vi "Trav_pos_global.vi"() -> ()   [LabVIEW 2010]
uses:
  Gen Trav/Traverse_cluster.ctl
  Gen Trav/Spacing.ctl
  Controls/Multi_run_mode.ctl
  Controls/Tunnel_Coordinates.ctl
panel:
  in  "Repeat Rows?":bool
  in  "Pause Until Seconds 1904":dbl
  in  "FFID Background":T1 {"Row Duration (mins)" format="%#.1f"; "Row No" min=0; "Trace Gas Concentration (%)" min=0.0 format="%#.2f"; "Emission Rate (l/min)" format="%#.2f"; "Tunnel Speed" format="%#.2f"; "Start X" format="%#.2f"; "Start Y" format="%#.2f"; "Start Z" format="%#.2f"; "End X" format="%#.2f"; "End Y" format="%#.2f"; "End Z" format="%#.2f"; "Averaging time (min)" min=0.0 format="%#.1f"}
  in  "Meas Setup Number":i32
  in  "Current Meas Setup File":string
  in  "Default Traverse Setup":string
  out "Simulation Time":timestamp
  out "Row completion times":timestamp[](array[timestamp])
  in  "Dummy Measurement?":bool
  in  "Jumped Positions":dbl[][](array[numeric])
  in  "Jump Bad Positions?":bool
  in  "Model Rotation (deg)":dbl format="%.2f"
  in  "Work in Tunnel Coordinates?":T4
  in  "Show User Metadata on Launch?":bool=TRUE
  in  "Measurement setup files":string[](array[string])
  out "Live Traverse Preview?":bool
  in  "Paused During Row?":bool
  in  "Speed Factor":dbl=1.0 min=0.1 max=5.0 format="%.2f"
  in  "Estimated Completion time":string
  in  "Start of Row time (Sec)":dbl
  out "Currently on point":i32=9
  in  "Current Row":T1 {"Row Duration (mins)" format="%#.1f"; "Row No" min=0; "Trace Gas Concentration (%)" min=0.0 format="%#.2f"; "Emission Rate (l/min)" format="%#.2f"; "Tunnel Speed" format="%#.2f"; "Start X" format="%#.2f"; "Start Y" format="%#.2f"; "Start Z" format="%#.2f"; "End X" format="%#.2f"; "End Y" format="%#.2f"; "End Z" format="%#.2f"; "Averaging time (min)" min=0.0 format="%#.1f"}
  in  "Source Control?":bool
  in  "Top level setup filename":path
  in  "Pause Acquisition":bool
  out "Axis Traversed":enum16{"X traverse", "Y traverse", "Z traverse"}(ring)
  in  "Traverse position":dbl[](array[numeric])=[0.0, 0.0, 0.0] format="%.2f"
  in  "Present Probe Positions":T5(array[cluster]) {"Z" format="%.1f"; "Y" format="%.1f"; "X" format="%.1f"}
  # "X                Y                   Z"
  # "X           Y            Z"
  # "Start"
  # "End"
  # "X           Y            Z"
  # "Start"
  # "End"
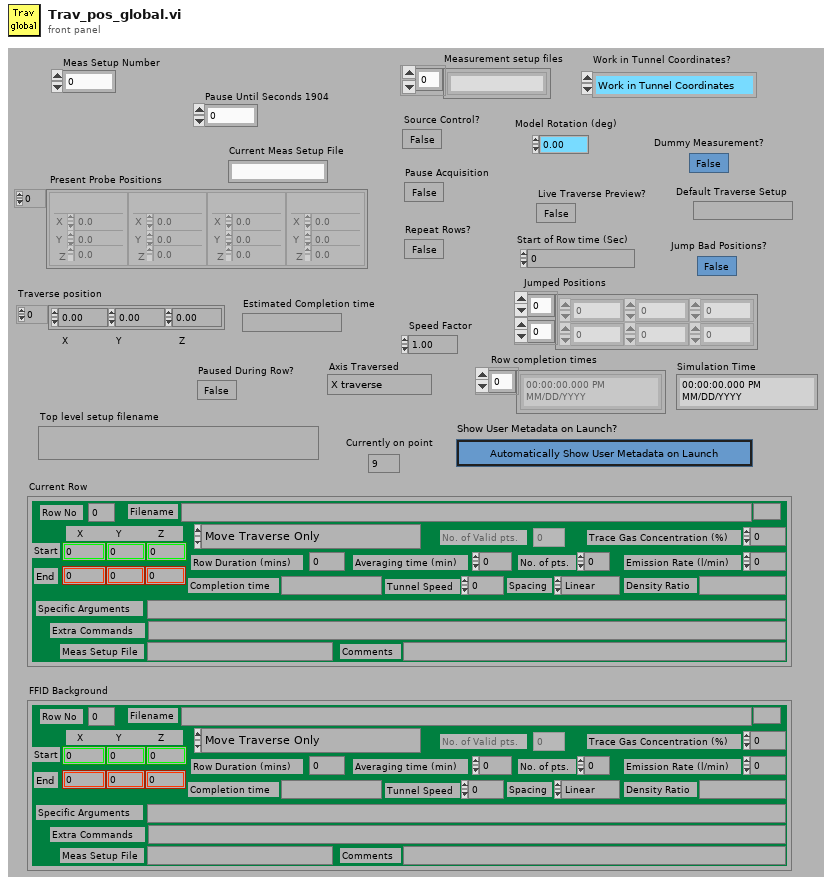
[diagram p1: front panel]
types:
  T1 = typedef "Traverse_cluster.ctl" = cluster{"Start X":dbl, "Start Y":dbl, "Start Z":dbl, "End X":dbl, "End Y":dbl, "End Z":dbl, "No. of pts.":i32, "Spacing":T2, "Filename":path, "Tunnel Speed":dbl, "Averaging time (min)":dbl, "Extra Commands":string, "Specific Arguments":string, "Emission Rate (l/min)":dbl, "Trace Gas Concentration (%)":dbl, "Density Ratio":string, "Comments":string, "Row No":i32, "Row Type Selector":T3, "Completion time":string, "Row Duration (mins)":dbl, "No. of Valid pts.":i32, "Meas Setup File":string}
  T2 = typedef "Spacing.ctl" = enum16{"Linear", "Log", "Gauss", "Specified", "N/A"}
  T3 = typedef "Multi_run_mode.ctl" = enum16{"Move Traverse Only", "Set Tunnel Speed Only", "Set Source Only", "Set Measurement Conditions", "Single Measurement", "Vertical Profile", "Lateral Profile", "Longitudinal Profile", "Explore Volume", "Multi-Axis Profile", "Auto Calibrate", "Meas Fast FID Bkgnd", "Check Beam Power", "Scanning Valve Measurement", "Run VI Named:", "Set ADAM Ch", "Wait (minutes)", "Send Message", "Synchronize With:", "Fall Back to this Row", "Turn Off Row Repeating", "Blank Row"}
  T4 = typedef "Tunnel_Coordinates.ctl" = enum16{"Work in Tunnel Coordinates", "Work in Model Coordinates"}
  T5 = cluster{"Name":string, "X":dbl, "Y":dbl, "Z":dbl}[]
diagram:
